vi "Two Lambda ZUP Control and Monitor.vi"() -> ()   [LabVIEW 2014]
uses:
  <vilib>/Instr/_visa.llb/VISA Configure Serial Port (Instr).vi
panel:
  in  "stop":bool
  out "ON/OFF-2":bool
  in  "Output ON/OFF-2":bool
  in  "Set Voltage-2":dbl min=0.0 max=19.9 step=0.1
  in  "Set Current-2":dbl min=0.0 max=9.9 step=0.1
  out "Output Voltage-2":dbl
  out "Output Current-2":dbl
  out "ON/OFF-1":bool
  in  "Output ON/OFF-1":bool
  in  "Set Voltage-1":dbl min=0.0 max=19.9 step=0.01
  in  "Set Current-1":dbl min=0.0 max=9.9 step=0.001
  out "Output Voltage-1":dbl
  out "Output Current-1":dbl
  in  "VISA resource name":refnum<visa-resource-name>
  # "ADD-1"
  # "ADD-2"
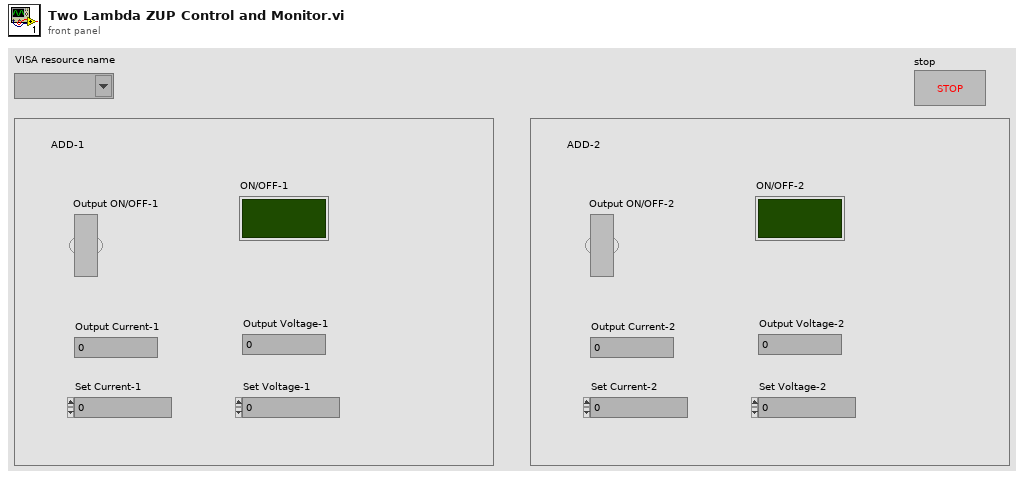
[diagram p1: front panel]
types:
  T1 = enum16{"Sets the power supply address-1", "Returns followed by the output On/Off status-1", "Returns the string AA (Actual Amper)-1", "Returns the string AV (Actual Voltage)-1", "Sets the power supply address-2", "Returns followed by the output On/Off status-2", "Returns the string AA (Actual Amper)-2", "Returns the string AV (Actual Voltage)-2"}
  T2 = enum16{"Output ON/OFF-1", "Set Current-1", "Set Voltage-1", "Output ON/OFF-2", "Set Current-2", "Set Voltage-2"}
  T3 = enum16{"Sets the power supply address", "Clears the communication buffer and the following registers", "Sets the power supply to local or remote mode", "Returns the remote/local setting", "Returns the power supply model identification", "Returns the software version", "Sets the output voltage value", "Returns the string SV (Set Voltage)", "Returns the string AV (Actual Voltage)", "Sets the output current in Ampers", "Returns the string SA (Set Amper)", "Returns the string AA (Actual Amper)", "Sets the output to On or Off", "Returns followed by the output On/Off status", "Sets the Foldback protection to On or Off", "Returns FD followed by the Foldback protection status", "Sets the over-voltage protection level in volts", "Returns the string OP  over-voltage protection value", "Sets the under-voltage protection limits in volts", "Returns the string UP under-voltage protection value", "Sets the auto-restart mode to On or Off", "Returns the string AS auto-restart mode status"}
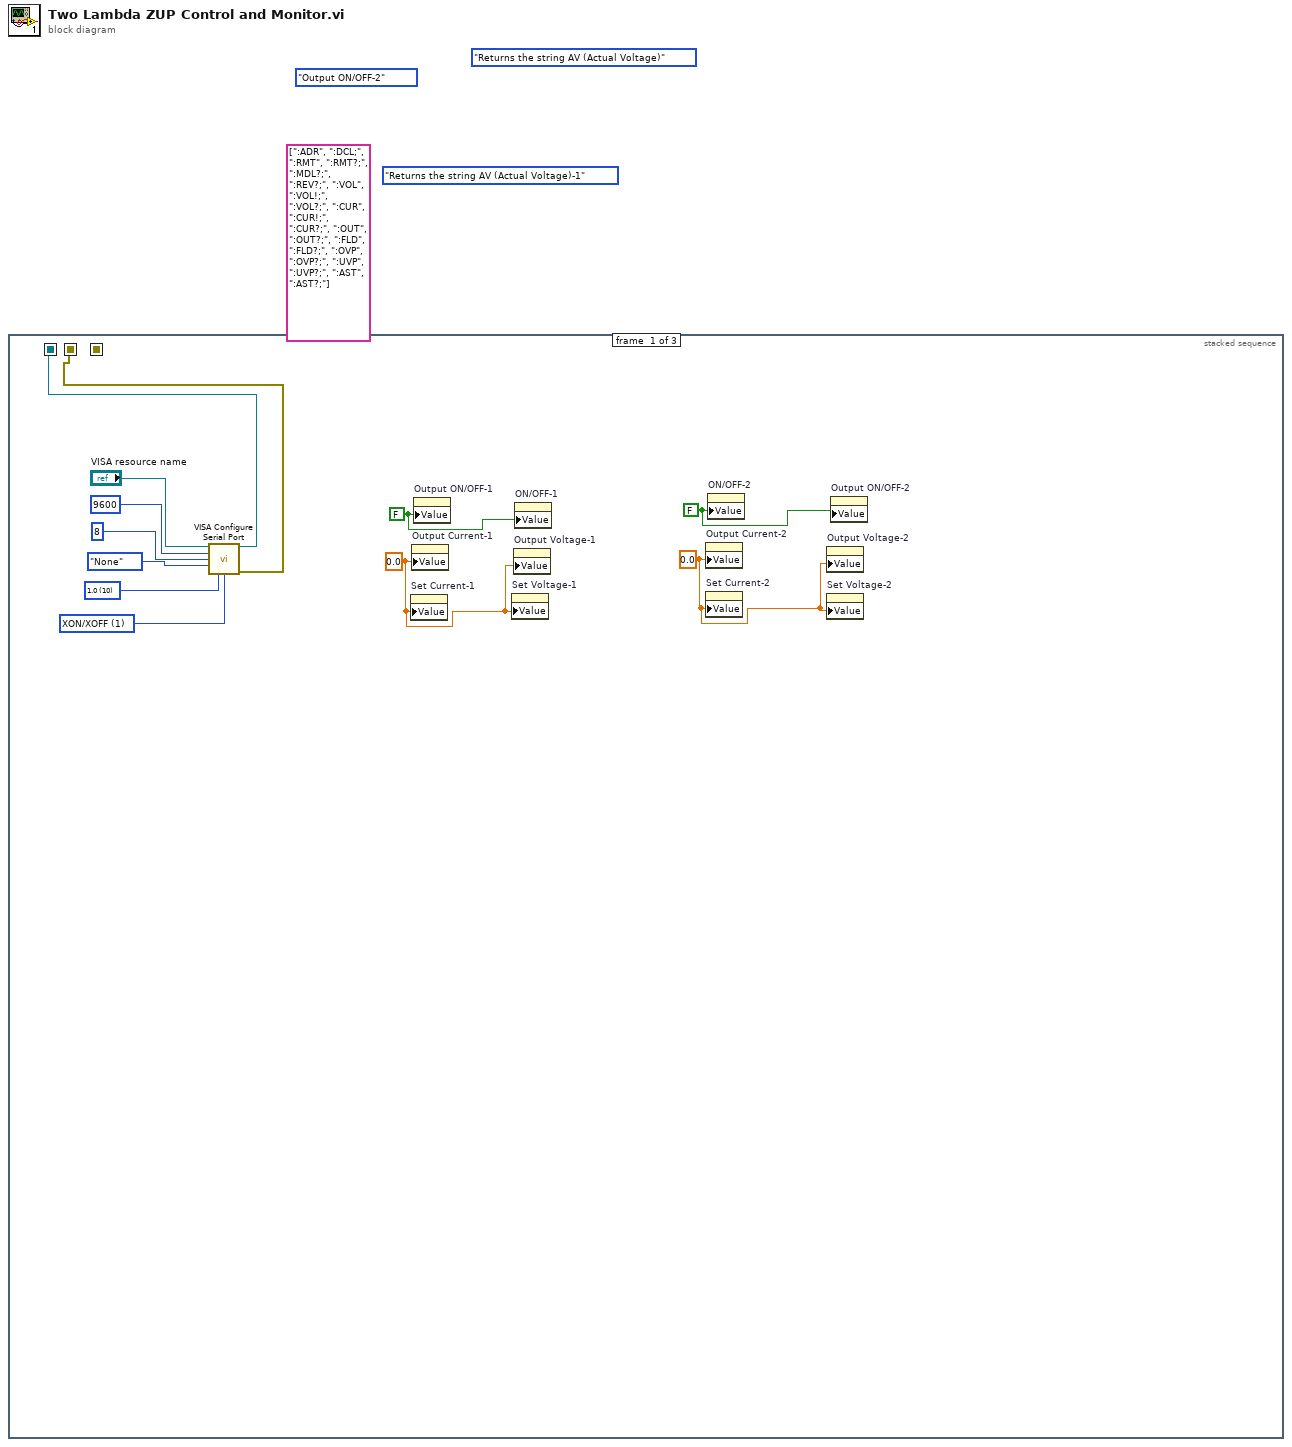
[diagram p0: block diagram]
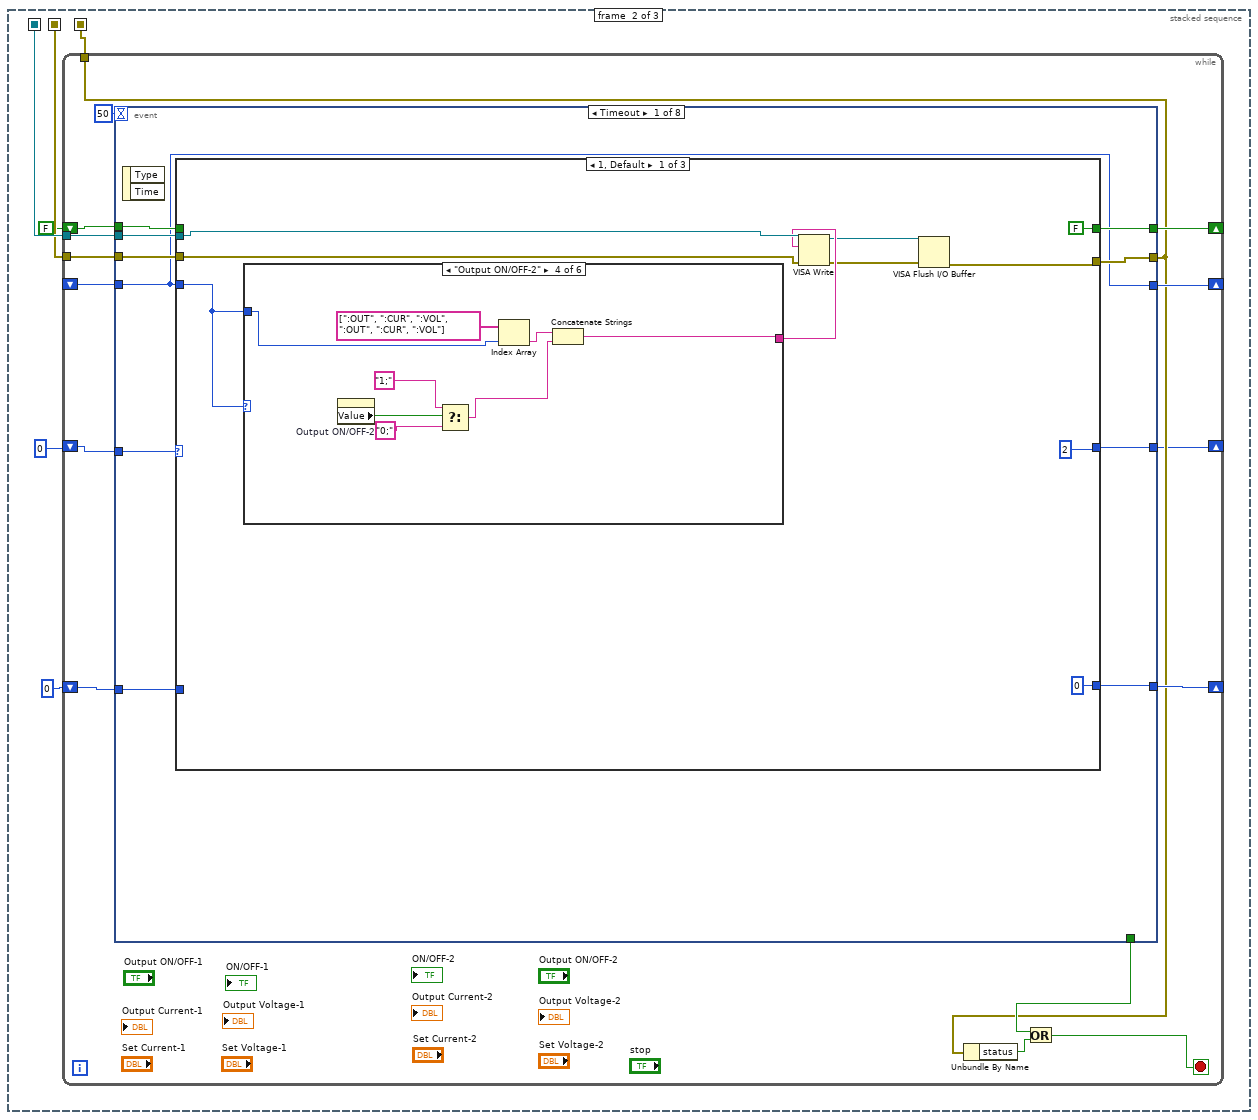
[diagram p2: hidden frame]
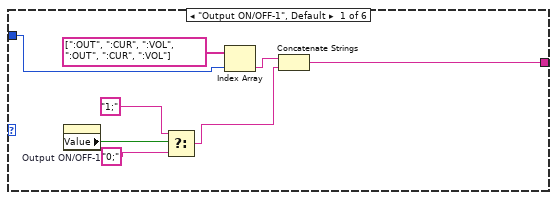
[diagram p3: hidden frame]
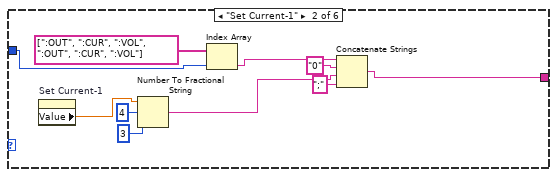
[diagram p4: hidden frame]
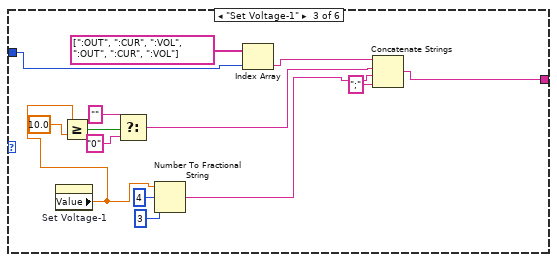
[diagram p5: hidden frame]
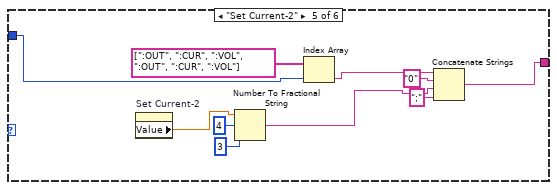
[diagram p6: hidden frame]
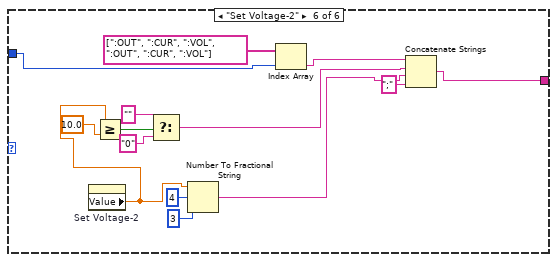
[diagram p7: hidden frame]
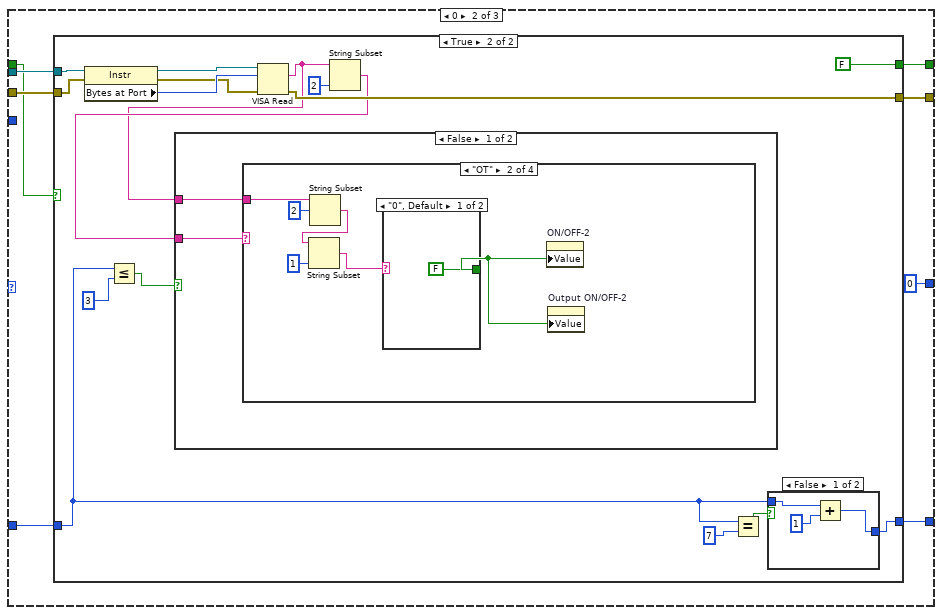
[diagram p8: hidden frame]
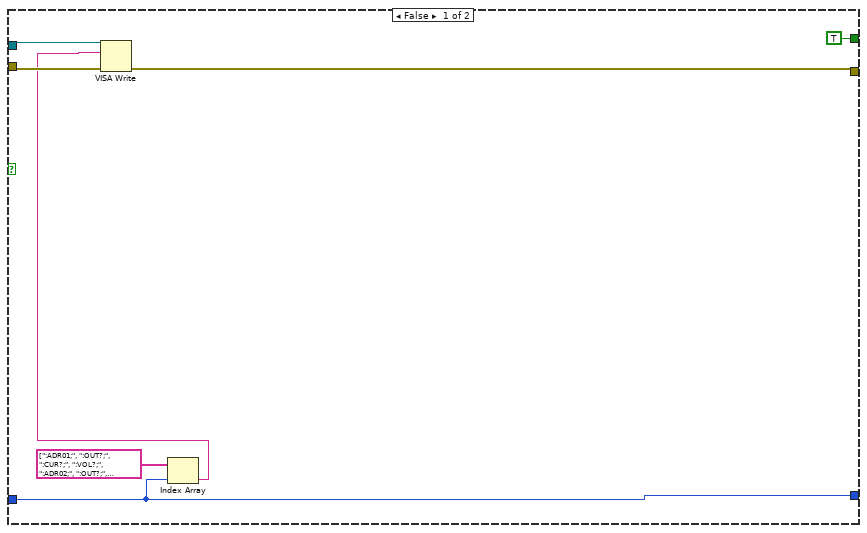
[diagram p9: hidden frame]
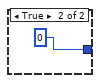
[diagram p10: hidden frame]
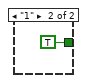
[diagram p12: hidden frame]
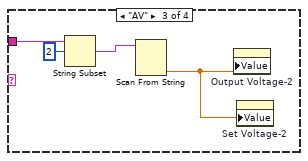
[diagram p13: hidden frame]
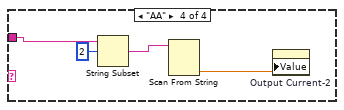
[diagram p14: hidden frame]
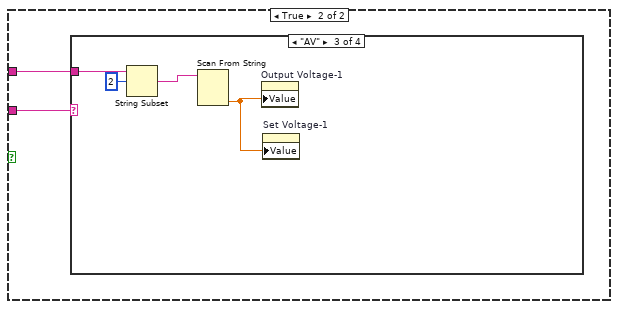
[diagram p15: hidden frame]
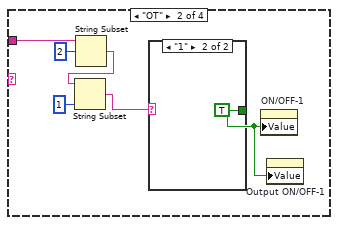
[diagram p17: hidden frame]
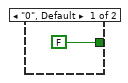
[diagram p18: hidden frame]
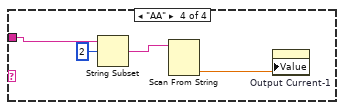
[diagram p19: hidden frame]
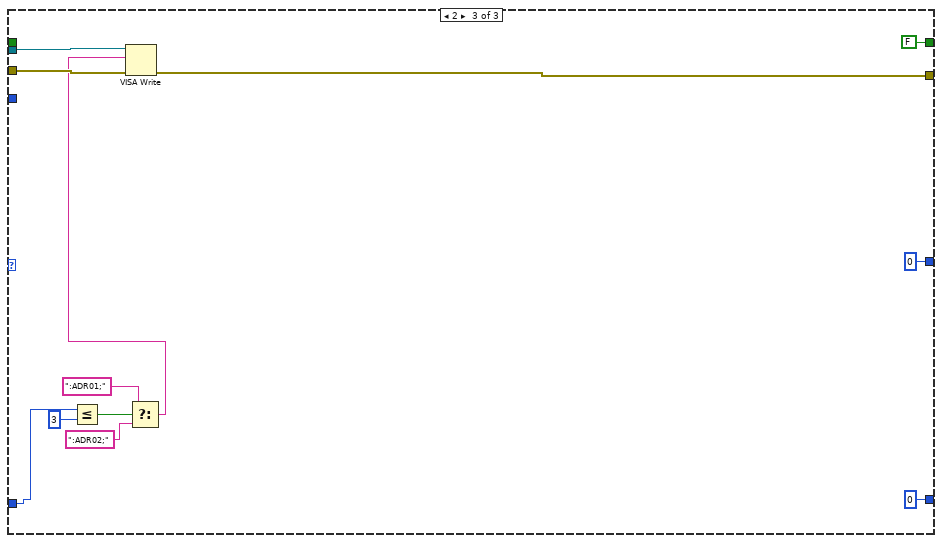
[diagram p20: hidden frame]
diagram:
  (unwired) T1."Returns the string AV (Actual Voltage)-1"
  (unwired) T2."Output ON/OFF-2" ("Enum")
  (unwired) string[] [":ADR", ":DCL;", ":RMT", ":RMT?;", ":MDL?;", ":REV?;", ":VOL", ":VOL!;", ":VOL?;", ":CUR", ":CUR!;", ":CUR?;", ":OUT", ":OUT?;", ":FLD", ":FLD?;", ":OVP", ":OVP?;", ":UVP", ":UVP?;", ":AST", ":AST?;"]
  (unwired) T3."Returns the string AV (Actual Voltage)" ("Command 1")
  n1 = stacked-sequence {
    seq-local: [w2 _ _] -> [_ w17 w275]
    seq-local: [w1 _ _] -> [_ w16 _]
    seq-local: [_ w14 _] -> [_ _ w274]
    frame #0 {
      w3 = 0.0 ("Output Current-2")
      w4 = FALSE ("Output ON/OFF-2")
      w5 = 0.0 ("Output Current-1")
      w6 = FALSE ("Output ON/OFF-1")
      w12 = u16 1 items=["None", "XON/XOFF", "RTS/CTS", "XON/XOFF & RTS/CTS", "DTR/DSR", "XON/XOFF & DTR/DSR"] ("flow control (0:none)")
      w11 = u16 10 items=["1.0"=10, "1.5"=15, "2.0"=20] ("stop bits (10: 1 bit)")
      n2 = call-poly "VISA Configure Serial Port"("VISA resource name"="VISA resource name", "baud rate (9600)"=u32 9600, "data bits (8)"=u16 8, "parity (0:none)"=enum16{"None", "Odd", "Even", "Mark", "Space"}."None", "stop bits (10: 1 bit)"=w11, "flow control (0:none)"=w12) -> ("VISA resource name out"=w2:refnum<visa-resource-name>, "error out"=w1:errorcluster)  [unwired: 8 in]
      n3 = property on="Set Current-1" class="DigNum (strict)"("Value"=w5) -> ()  [unwired: 2 in, 2 out]
      n4 = property on="Output Current-1" class="DigNum (strict)"("Value"=w5) -> ()  [unwired: 2 in, 2 out]
      n5 = property on="Output ON/OFF-1" class="Bool (strict)"("Value"=w6) -> ()  [unwired: 2 in, 2 out]
      n6 = property on="Set Voltage-1" class="DigNum (strict)"("Value"=w5) -> ()  [unwired: 2 in, 2 out]
      n7 = property on="Output Voltage-1" class="DigNum (strict)"("Value"=w5) -> ()  [unwired: 2 in, 2 out]
      n8 = property on="ON/OFF-1" class="Bool (strict)"("Value"=w6) -> ()  [unwired: 2 in, 2 out]
      n9 = property on="Output Current-2" class="DigNum (strict)"("Value"=w3) -> ()  [unwired: 2 in, 2 out]
      n10 = property on="Set Current-2" class="DigNum (strict)"("Value"=w3) -> ()  [unwired: 2 in, 2 out]
      n11 = property on="ON/OFF-2" class="Bool (strict)"("Value"=w4) -> ()  [unwired: 2 in, 2 out]
      n12 = property on="Output Voltage-2" class="DigNum (strict)"("Value"=w3) -> ()  [unwired: 2 in, 2 out]
      n13 = property on="Set Voltage-2" class="DigNum (strict)"("Value"=w3) -> ()  [unwired: 2 in, 2 out]
      n14 = property on="Output ON/OFF-2" class="Bool (strict)"("Value"=w4) -> ()  [unwired: 2 in, 2 out]
    }
    frame #1 {
      n15 = while {
        shift-right: [w31] -> _
        shift-left: 0 -> [w32]
        tunnel: w17 -> [w30]
        tunnel: w16 -> [w29]
        shift-right: [w25] -> _
        shift-left: FALSE -> [w24]
        shift-right: [w19] -> _
        shift-left: 0 -> [w23]
        shift-right: [w22] -> _
        shift-left: _ -> [w21]
        tunnel: [w20] -> w14
        stop <- w26 stop-if-true
        n16 = event shown="[0] Timeout" {
          selector: _ -> [_ _ _ _ _ _ _ _]
          dyn-events: _ -> [_ _ _ _ _ _ _ _]
          timeout: 50 -> [_ _ _ _ _ _ _ _]
          tunnel: w32 -> [w37 w207 w218 w229 w240 w251 w262 w268]
          tunnel: [w38 w207 w218 w229 w240 w251 w262 w268] -> w31
          tunnel: [_ _ _ _ _ _ _ TRUE] -> w28
          tunnel: w30 -> [w43 w204 w215 w226 w237 w248 w259 _]
          tunnel: w29 -> [w42 w203 w214 w225 w236 w247 w258 w270]
          tunnel: [w41 w211 w221 w232 w243 w254 w265 w270] -> w20
          tunnel: [w40 w208 w219 w230 w241 w252 w263 w271] -> w25
          tunnel: w24 -> [w39 w208 w219 w230 w241 w252 w263 w271]
          tunnel: w23 -> [w35 _ _ _ _ _ _ w267]
          tunnel: [w36 T2."Output ON/OFF-1" ("Enum") T2."Set Voltage-1" ("Enum") T2."Set Current-1" ("Enum") T2."Output ON/OFF-2" ("Enum") T2."Set Voltage-2" ("Enum") T2."Set Current-2" ("Enum") w269] -> w22
          tunnel: w21 -> [w36 _ _ _ _ _ _ w269]
          tunnel: [w34 1 1 1 1 1 1 w267] -> w19
          event Timeout {
            n17 = event-data() -> ()  [unwired: 1 in, 2 out]
            n18 = case shown="1, Default" w35 {
              tunnel: w43 -> [w52 w125 w199]
              tunnel: w42 -> [w51 w124 w198]
              tunnel: [w46 w123 w191] -> w41
              tunnel: [FALSE w122 FALSE] -> w40
              tunnel: w39 -> [_ w121 _]
              tunnel: [0 w120 0] -> w38
              tunnel: w37 -> [_ w119 w197]
              tunnel: [2 0 0] -> w34
              tunnel: w36 -> [w53 _ _]
              frame 1, Default {
                n19 = case shown="\"Output ON/OFF-2\"" w53 {
                  tunnel: w53 -> [w61 w70 w79 w87 w95 w105]
                  tunnel: [w54 w62 w76 w86 w94 w104] -> w50
                  frame "Output ON/OFF-1", Default {
                    n20 = property on="Output ON/OFF-1" class="Bool (strict)"() -> ("Value"=w59:bool)  [unwired: 2 in, 2 out]
                    n21 = Select(t="1;", s=w59, f="0;") -> (s? t:f=w55:string)
                    n22 = Index Array(array=string[] [":OUT", ":CUR", ":VOL", ":OUT", ":CUR", ":VOL"], index=w61) -> (element=w56:string)
                    n23 = Concatenate Strings(w56, w55) -> (w54:string)
                  }
                  frame "Set Current-1" {
                    n24 = property on="Set Current-1" class="DigNum (strict)"() -> ("Value"=w67:dbl)  [unwired: 2 in, 2 out]
                    n25 = Number To Fractional String(number=w67, width (-)=i16 4, precision (6)=i16 3) -> (F-format string=w64:string)  [unwired: 1 in]
                    n26 = Index Array(array=string[] [":OUT", ":CUR", ":VOL", ":OUT", ":CUR", ":VOL"], index=w70) -> (element=w66:string)
                    n27 = Concatenate Strings(w66, "0" ("string"), w64, ";" ("string")) -> (w62:string)
                  }
                  frame "Set Voltage-1" {
                    n28 = property on="Set Voltage-1" class="DigNum (strict)"() -> ("Value"=w74:dbl)  [unwired: 2 in, 2 out]
                    n29 = Greater Or Equal?(x=w74, y=10.0 ("x")) -> (x >= y?=w78:bool)
                    n30 = Select(t="", s=w78, f="0" ("string")) -> (s? t:f=w77:string)
                    n31 = Number To Fractional String(number=w74, width (-)=i16 4, precision (6)=i16 3) -> (F-format string=w81:string)  [unwired: 1 in]
                    n32 = Index Array(array=string[] [":OUT", ":CUR", ":VOL", ":OUT", ":CUR", ":VOL"], index=w79) -> (element=w82:string)
                    n33 = Concatenate Strings(w82, w77, w81, ";" ("string")) -> (w76:string)
                  }
                  frame "Output ON/OFF-2" {
                    n34 = property on="Output ON/OFF-2" class="Bool (strict)"() -> ("Value"=w92:bool)  [unwired: 2 in, 2 out]
                    n35 = Select(t="1;", s=w92, f="0;") -> (s? t:f=w88:string)
                    n36 = Index Array(array=string[] [":OUT", ":CUR", ":VOL", ":OUT", ":CUR", ":VOL"], index=w87) -> (element=w89:string)
                    n37 = Concatenate Strings(w89, w88) -> (w86:string)
                  }
                  frame "Set Current-2" {
                    n38 = property on="Set Current-2" class="DigNum (strict)"() -> ("Value"=w100:dbl)  [unwired: 2 in, 2 out]
                    n39 = Number To Fractional String(number=w100, width (-)=i16 4, precision (6)=i16 3) -> (F-format string=w97:string)  [unwired: 1 in]
                    n40 = Index Array(array=string[] [":OUT", ":CUR", ":VOL", ":OUT", ":CUR", ":VOL"], index=w95) -> (element=w99:string)
                    n41 = Concatenate Strings(w99, "0" ("string"), w97, ";" ("string")) -> (w94:string)
                  }
                  frame "Set Voltage-2" {
                    n42 = property on="Set Voltage-2" class="DigNum (strict)"() -> ("Value"=w108:dbl)  [unwired: 2 in, 2 out]
                    n43 = Greater Or Equal?(x=w108, y=10.0 ("x")) -> (x >= y?=w111:bool)
                    n44 = Select(t="", s=w111, f="0" ("string")) -> (s? t:f=w110:string)
                    n45 = Number To Fractional String(number=w108, width (-)=i16 4, precision (6)=i16 3) -> (F-format string=w113:string)  [unwired: 1 in]
                    n46 = Index Array(array=string[] [":OUT", ":CUR", ":VOL", ":OUT", ":CUR", ":VOL"], index=w105) -> (element=w114:string)
                    n47 = Concatenate Strings(w114, w110, w113, ";" ("string")) -> (w104:string)
                  }
                }
                n48 = VISA Write(VISA resource name=w52, write buffer=w50, error in (no error)=w51) -> (VISA resource name out=w48:refnum<visa-resource-name>, error out=w47:errorcluster)  [unwired: 1 out]
                n49 = VISA Flush I/O Buffer(VISA resource name=w48, error in (no error)=w47) -> (error out=w46:errorcluster)  [unwired: 1 in, 1 out]
              }
              frame 0 {
                n50 = case shown="True" w121 {
                  tunnel: w125 -> [w132 w144]
                  tunnel: w124 -> [w131 w143]
                  tunnel: [w130 w142] -> w123
                  tunnel: [TRUE FALSE] -> w122
                  tunnel: [w126 w134] -> w120
                  tunnel: w119 -> [w126 w133]
                  frame False {
                    n51 = Index Array(array=string[] [":ADR01;", ":OUT?;", ":CUR?;", ":VOL?;", ":ADR02;", ":OUT?;", ":CUR?;", ":VOL?;"], index=w126) -> (element=w127:string)
                    n52 = VISA Write(VISA resource name=w132, write buffer=w127, error in (no error)=w131) -> (error out=w130:errorcluster)  [unwired: 2 out]
                  }
                  frame True {
                    n53 = property class="Instr"(reference=w144, error in=w143) -> (reference out=w147:refnum<visa-resource-name>, error out=w145:errorcluster, "Bytes at Port"=w146:u32)
                    n54 = Less Or Equal?(x=w133, y=3 ("upper limit")) -> (x <= y?=w138:bool)
                    n55 = VISA Read(VISA resource name=w147, byte count=w146, error in (no error)=w145) -> (read buffer=w139:string, error out=w142:errorcluster)  [unwired: 2 out]
                    n56 = String Subset(string=w139, length (rest)=2 ("length (rest)")) -> (substring=w140:string)  [unwired: 1 in]
                    n57 = case shown="False" w138 {
                      tunnel: w140 -> [w153 w172]
                      tunnel: w139 -> [w154 w171]
                      frame False {
                        n58 = case shown="\"OT\"" w153 {
                          tunnel: w154 -> [_ w160 w166 w168]
                          frame "False", Default {
                          }
                          frame "OT" {
                            n59 = String Subset(string=w160, offset (0)=2) -> (substring=w158:string)  [unwired: 1 in]
                            n60 = String Subset(string=w158, length (rest)=1 ("length (rest)")) -> (substring=w156:string)  [unwired: 1 in]
                            n61 = case shown="\"0\", Default" w156 {
                              tunnel: [FALSE ("Output ON/OFF-1") TRUE ("Output ON/OFF-1")] -> w155
                              frame "0", Default {
                              }
                              frame "1" {
                              }
                            }
                            n62 = property on="ON/OFF-2" class="Bool (strict)"("Value"=w155) -> ()  [unwired: 2 in, 2 out]
                            n63 = property on="Output ON/OFF-2" class="Bool (strict)"("Value"=w155) -> ()  [unwired: 2 in, 2 out]
                          }
                          frame "AV" {
                            n64 = String Subset(string=w166, offset (0)=2) -> (substring=w164:string)  [unwired: 1 in]
                            n65 = Scan From String(input string=w164) -> (output 1=w163:dbl)  [unwired: 4 in, 3 out]
                            n66 = property on="Output Voltage-2" class="DigNum (strict)"("Value"=w163) -> ()  [unwired: 2 in, 2 out]
                            n67 = property on="Set Voltage-2" class="DigNum (strict)"("Value"=w163) -> ()  [unwired: 2 in, 2 out]
                          }
                          frame "AA" {
                            n68 = String Subset(string=w168, offset (0)=2) -> (substring=w169:string)  [unwired: 1 in]
                            n69 = Scan From String(input string=w169) -> (output 1=w167:dbl)  [unwired: 4 in, 3 out]
                            n70 = property on="Output Current-2" class="DigNum (strict)"("Value"=w167) -> ()  [unwired: 2 in, 2 out]
                          }
                        }
                      }
                      frame True {
                        n71 = case shown="\"AV\"" w172 {
                          tunnel: w171 -> [_ w178 w184 w186]
                          frame "False", Default {
                          }
                          frame "OT" {
                            n72 = String Subset(string=w178, offset (0)=2) -> (substring=w176:string)  [unwired: 1 in]
                            n73 = String Subset(string=w176, length (rest)=1 ("length (rest)")) -> (substring=w174:string)  [unwired: 1 in]
                            n74 = case shown="\"1\"" w174 {
                              tunnel: [FALSE ("Output ON/OFF-1") TRUE ("Output ON/OFF-1")] -> w173
                              frame "0", Default {
                              }
                              frame "1" {
                              }
                            }
                            n75 = property on="ON/OFF-1" class="Bool (strict)"("Value"=w173) -> ()  [unwired: 2 in, 2 out]
                            n76 = property on="Output ON/OFF-1" class="Bool (strict)"("Value"=w173) -> ()  [unwired: 2 in, 2 out]
                          }
                          frame "AV" {
                            n77 = String Subset(string=w184, offset (0)=2) -> (substring=w182:string)  [unwired: 1 in]
                            n78 = Scan From String(input string=w182) -> (output 1=w181:dbl)  [unwired: 4 in, 3 out]
                            n79 = property on="Output Voltage-1" class="DigNum (strict)"("Value"=w181) -> ()  [unwired: 2 in, 2 out]
                            n80 = property on="Set Voltage-1" class="DigNum (strict)"("Value"=w181) -> ()  [unwired: 2 in, 2 out]
                          }
                          frame "AA" {
                            n81 = String Subset(string=w186, offset (0)=2) -> (substring=w187:string)  [unwired: 1 in]
                            n82 = Scan From String(input string=w187) -> (output 1=w185:dbl)  [unwired: 4 in, 3 out]
                            n83 = property on="Output Current-1" class="DigNum (strict)"("Value"=w185) -> ()  [unwired: 2 in, 2 out]
                          }
                        }
                      }
                    }
                    n84 = Equal?(x=w133, y=7) -> (x = y?=w135:bool)
                    n85 = case shown="False" w135 {
                      tunnel: [w149 0] -> w134
                      tunnel: w133 -> [w151 _]
                      frame False {
                        n86 = Add(x=w151, y=1) -> (x+y=w149:i32)
                      }
                      frame True {
                      }
                    }
                  }
                }
              }
              frame 2 {
                n87 = Less Or Equal?(x=w197, y=3) -> (x <= y?=w195:bool)
                n88 = Select(t=":ADR01;" ("write buffer"), s=w195, f=":ADR02;" ("write buffer")) -> (s? t:f=w192:string)
                n89 = VISA Write(VISA resource name=w199, write buffer=w192, error in (no error)=w198) -> (error out=w191:errorcluster)  [unwired: 2 out]
              }
            }
          }
          event "Output ON/OFF-1": Value Change {
            n90 = event-data() -> ()  [unwired: 1 in, 6 out]
            n91 = VISA Flush I/O Buffer(VISA resource name=w204, error in (no error)=w203) -> (VISA resource name out=w202:refnum<visa-resource-name>, error out=w201:errorcluster)  [unwired: 1 in]
            n92 = VISA Write(VISA resource name=w202, write buffer=":ADR01;", error in (no error)=w201) -> (error out=w211:errorcluster)  [unwired: 2 out]
            n93 = Wait (ms)(milliseconds to wait=u32 50) -> ()  [unwired: 1 out]
          }
          event "Set Voltage-1": Value Change {
            n94 = event-data() -> ()  [unwired: 1 in, 6 out]
            n95 = VISA Flush I/O Buffer(VISA resource name=w215, error in (no error)=w214) -> (VISA resource name out=w213:refnum<visa-resource-name>, error out=w212:errorcluster)  [unwired: 1 in]
            n96 = VISA Write(VISA resource name=w213, write buffer=":ADR01;", error in (no error)=w212) -> (error out=w221:errorcluster)  [unwired: 2 out]
            n97 = Wait (ms)(milliseconds to wait=u32 50) -> ()  [unwired: 1 out]
          }
          event "Set Current-1": Value Change {
            n98 = event-data() -> ()  [unwired: 1 in, 6 out]
            n99 = VISA Flush I/O Buffer(VISA resource name=w226, error in (no error)=w225) -> (VISA resource name out=w224:refnum<visa-resource-name>, error out=w223:errorcluster)  [unwired: 1 in]
            n100 = VISA Write(VISA resource name=w224, write buffer=":ADR01;", error in (no error)=w223) -> (error out=w232:errorcluster)  [unwired: 2 out]
            n101 = Wait (ms)(milliseconds to wait=u32 50) -> ()  [unwired: 1 out]
          }
          event "Output ON/OFF-2": Value Change {
            n102 = event-data() -> ()  [unwired: 1 in, 6 out]
            n103 = VISA Flush I/O Buffer(VISA resource name=w237, error in (no error)=w236) -> (VISA resource name out=w235:refnum<visa-resource-name>, error out=w234:errorcluster)  [unwired: 1 in]
            n104 = VISA Write(VISA resource name=w235, write buffer=":ADR02;", error in (no error)=w234) -> (error out=w243:errorcluster)  [unwired: 2 out]
            n105 = Wait (ms)(milliseconds to wait=u32 50) -> ()  [unwired: 1 out]
          }
          event "Set Voltage-2": Value Change {
            n106 = event-data() -> ()  [unwired: 1 in, 6 out]
            n107 = VISA Flush I/O Buffer(VISA resource name=w248, error in (no error)=w247) -> (VISA resource name out=w246:refnum<visa-resource-name>, error out=w245:errorcluster)  [unwired: 1 in]
            n108 = VISA Write(VISA resource name=w246, write buffer=":ADR02;", error in (no error)=w245) -> (error out=w254:errorcluster)  [unwired: 2 out]
            n109 = Wait (ms)(milliseconds to wait=u32 50) -> ()  [unwired: 1 out]
          }
          event "Set Current-2": Value Change {
            n110 = event-data() -> ()  [unwired: 1 in, 6 out]
            n111 = VISA Flush I/O Buffer(VISA resource name=w259, error in (no error)=w258) -> (VISA resource name out=w257:refnum<visa-resource-name>, error out=w256:errorcluster)  [unwired: 1 in]
            n112 = VISA Write(VISA resource name=w257, write buffer=":ADR02;", error in (no error)=w256) -> (error out=w265:errorcluster)  [unwired: 2 out]
            n113 = Wait (ms)(milliseconds to wait=u32 50) -> ()  [unwired: 1 out]
          }
          event "stop": Mouse Down {
            n114 = event-data() -> ()  [unwired: 1 in, 7 out]
          }
        }
        n115 = Unbundle By Name(w20) -> ("status"=w27:bool)
        n116 = Or(x=w28, y=w27) -> (x .or. y?=w26:bool)
      }
    }
    frame #2 {
      n117 = VISA Close(VISA resource name=w275, error in (no error)=w274) -> (error out=w273:errorcluster)
      n118 = call <vilib>:"Simple Error Handler.vi"("error in (no error)"=w273) -> ()  [unwired: 4 in, 5 out]
    }
  }
